vi "Disable Controller.vi"(8 "error in (no error)":errorcluster, 10 "CAN Offset":u32 format="%x", 11 "interface object in":refnum<k20>) -> (0 "error out":errorcluster, 3 "interface object out":refnum<k20>)   [LabVIEW 2014]
uses:
  <vilib>/RioEmbeddedCAN/RioEmbeddedCAN.llb/CANFrameControl.ctl
  <vilib>/RioEmbeddedCAN/RioEmbeddedCAN.llb/CANWaitTransmitComplete.vi
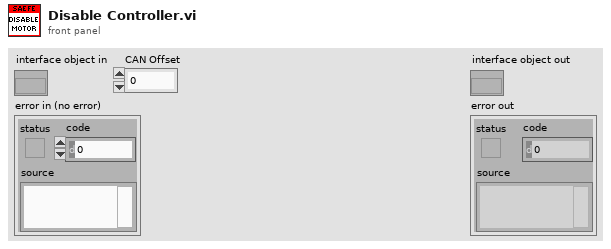
[diagram p1: front panel]
types:
  T1 = typedef "CANFrameControl.ctl" = cluster{"identifier":u32, "extended?":bool, "type":u8, "payload":u8[]}
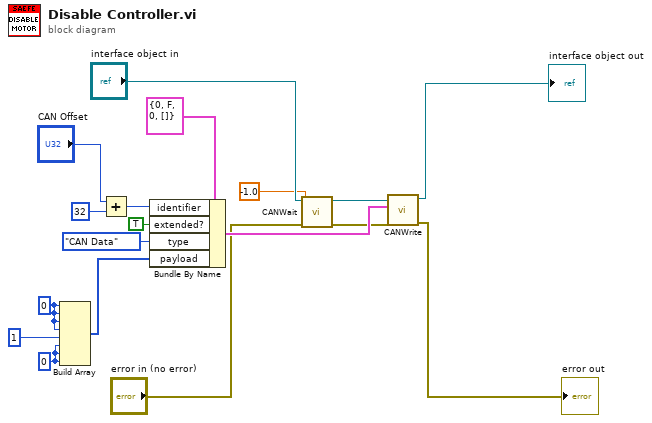
[diagram p0: block diagram]
diagram:
  w6 = u8 0 ("element")
  w8 = u8 0 ("element")
  n1 = Build Array(w8, w8, w8, w8, u8 1 ("element"), w6, w6, w6) -> (w10:u8[])
  n2 = Add(x="CAN Offset", y=u32 32) -> (x+y=w14:u32)
  n3 = Bundle By Name(cluster=T1 {"identifier"=0, "extended?"=FALSE, "type"=0, "payload"=[]} ("CAN frame"), "identifier"=w14, "extended?"=TRUE, "type"=enum8{"CAN Data", "CAN Remote"}."CAN Data", "payload"=w10) -> (w15:T1)
  n4 = call-poly <vilib>:"CANWait.vi"("error in (no error)"="error in (no error)", "timeout (0 s)"=-1.0, "interface object in"="interface object in") -> ("error out"=w4:errorcluster, "interface object out"=w5:refnum<k20>)  [unwired: 7 in]
  n5 = call <vilib>:"CANWrite.vi"("error in (no error)"=w4, "CAN frame"=w15, "interface object in"=w5) -> ("error out"=→"error out":errorcluster, "interface object out"=→"interface object out":refnum<k20>)  [unwired: 7 in]
